vi "Host Test1.vi"() -> ()   [LabVIEW 2012]
uses:
  <vilib>/FPGAPlugInAG/PCI-7831R/niLvFpga_Open_PCI-7831R.vi
  <vilib>/rvi/interface/common/dynamic/niFpgaDynamicAddResources.vi
  <vilib>/Utility/error.llb/Error Cluster From Error Code.vi
  <vilib>/rvi/errors/niLvFpgaAdjustHostInterfaceError.vi
  <vilib>/FPGAPlugInAG/Dynamic/niLvFpga_Close_Dynamic.vi
  <vilib>/rvi/interface/nirviOpenFPGA/nirviOpenFPGA.xnode
  SB130-XPS/Documents/FPGA-project-apporach-retraction/FPGA Bitfiles/Apporach-Retract_FPGATarget2_TargetTest_luhszpaEPZQ.lvbitx
  Target Test.vi
  <vilib>/rvi/interface/nirviReadWriteControl/nirviReadWriteControl.xnode
  <vilib>/rvi/interface/nirviCloseFPGA/nirviCloseFPGA.xnode
  NiFpgaLv.dll
  <vilib>/rvi/interface/Simulation/niFpgaSimulationCallBeginRW.vi
panel:
  in  "Digital Step":i32=640
  out "Control Voltage In Range":bool
  out "Control Voltage Host Indicator":i32
  in  "Control Voltage":i32
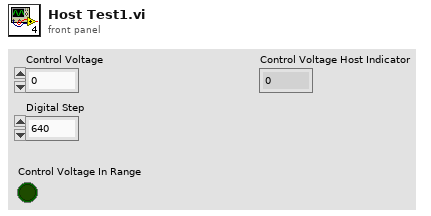
[diagram p1: front panel]
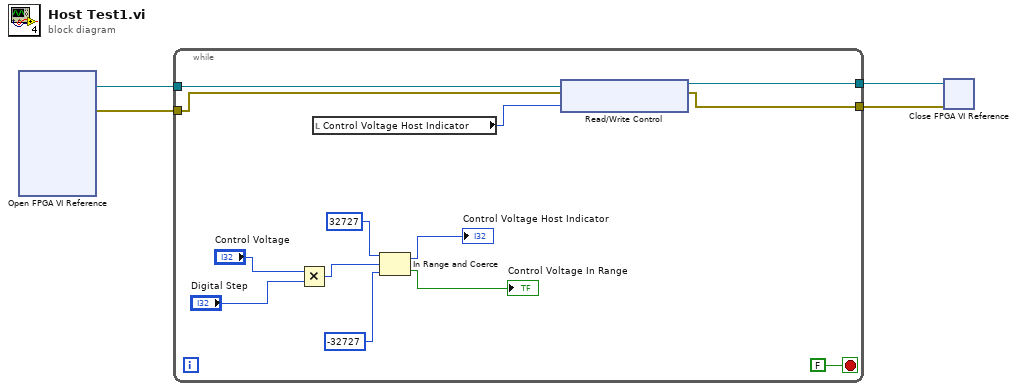
[diagram p0: block diagram]
diagram:
  n1 = xnode "Open FPGA VI Reference"() -> ("FPGA VI Reference Out"=w3:refnum<k20>, "error out"=w4:errorcluster)  [unwired: 2 in]
  n2 = while {
    tunnel: w3 -> [w9]
    tunnel: w4 -> [w8]
    tunnel: [w7] -> w2
    tunnel: [w6] -> w1
    stop <- FALSE stop-if-true
    n3 = Multiply(x="Control Voltage", y="Digital Step") -> (x*y=w14:i32)
    n4 = local read "Control Voltage Host Indicator"() -> (w5:i32)
    n5 = In Range and Coerce(upper limit=32727, x=w14, lower limit=-32727) -> (coerced(x)=→"Control Voltage Host Indicator":i32, In Range?=→"Control Voltage In Range":bool)
    n6 = xnode "Read/Write Control"("FPGA VI Reference In"=w9, "error in"=w8, "Host Output Voltage"=w5) -> ("FPGA VI Reference Out"=w7:refnum<k20>, "error out"=w6:errorcluster)
  }
  n7 = xnode "Close FPGA VI Reference"("FPGA VI Reference In"=w2, "error in"=w1) -> ()  [unwired: 1 out]
